vi "Data_filtering_speed_test.vi"() -> ()   [LabVIEW 2018]
uses:
  SubVi's/Controls/CTL_Filter_selector.ctl
  <vilib>/Analysis/NI_AALBase.lvlib
panel:
  out "0th order SG coefficients":dbl[](array[numeric])
  out "subarray":dbl[](array[numeric])
  in  "Filter type 3":u16(ring)=6 items=["None", "Kalman 0.50", "Kalman 0.30", "Kalman 0.12", "Savitzky-Golay 3/5", "Savitzky-Golay 3/11", "Savitzky-Golay 3/31"]
  out "Waveform Chart 3":T1(graph)
  in  "Filter type 2":T2={"Type"=1, "Length"=31, "Order"=3} {"Length" min=5 max=301 step=2; "Order" min=3 max=11 step=2; "Type" items=["None", "Savitzky-Golay"]}
  in  "Filter type":T2={"Type"=1, "Length"=31, "Order"=3} {"Length" min=5 max=301 step=2; "Order" min=3 max=11 step=2; "Type" items=["None", "Savitzky-Golay"]}
  out "standard deviation 2":dbl format="%0.2f"
  out "us per calc 2":dbl format="%0.2f"
  out "Calc time histogram 2":T3(graph)
  out "Waveform Chart 2":cluster{"Filtered sample":dbl, "X1":sgl}(graph)
  out "standard deviation":dbl format="%0.2f"
  out "us per calc":dbl format="%0.2f"
  out "Calc time histogram":T3(graph)
  out "Waveform Chart":cluster{"X1 filtered":dbl, "X1 raw":dbl}(graph)
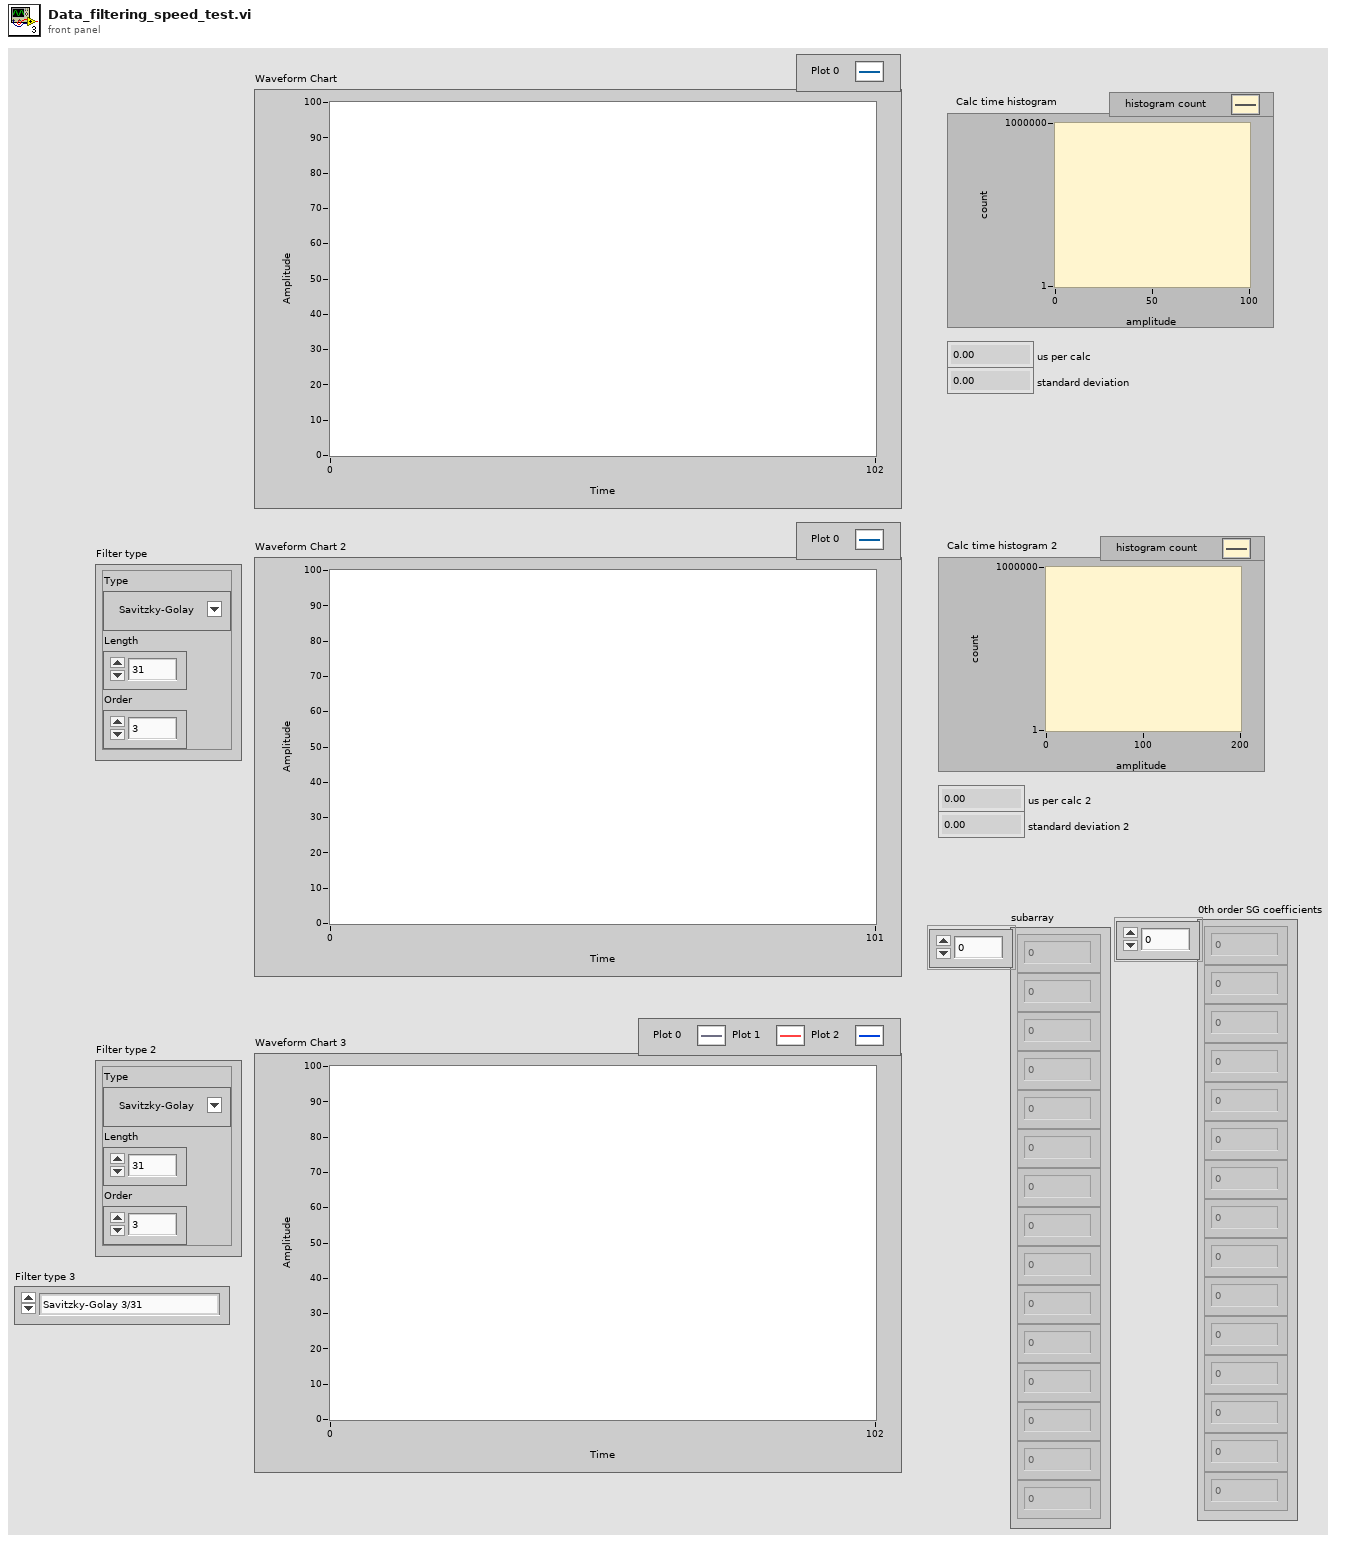
[diagram p1: front panel]
types:
  T1 = cluster{"X1 raw":dbl, "X1 filtered":dbl, "Filtered sample":dbl}
  T2 = typedef "CTL_Filter_selector.ctl" = cluster{"Type":u16, "Length":i32, "Order":i32}
  T3 = cluster{"X Values":dbl[], "Histogram: h(x)":i32[]}
  T4 = cluster{"SG coefficients 3/5":cluster{"0th order SG coefficients":dbl[], "1st order SG coefficients":dbl[]}, "SG coefficients 3/11":cluster{"0th order SG coefficients":dbl[], "1st order SG coefficients":dbl[]}, "SG coefficients 3/31":cluster{"0th order SG coefficients":dbl[], "1st order SG coefficients":dbl[]}, "SG coefficients 3/51":cluster{"0th order SG coefficients":dbl[], "1st order SG coefficients":dbl[]}}
  T5 = cluster{"0th order SG coefficients":dbl[], "1st order SG coefficients":dbl[]}
  T6 = cluster{"ms since ON":u32, "delta time":u32, "X1":sgl, "Y1":sgl, "X2":sgl, "Y2":sgl, "TTL in 1":i16, "TTL in 2":i16, "Frame timestamp":timestamp, "Frame OK":bool}
  T7 = cluster{"Filtered sample":dbl, "Filtered sample":dbl, "Filtered sample":dbl, "Filtered sample":dbl}
  T8 = cluster{"X1 filtered":dbl, "Y1 filtered":dbl, "X2 filtered":dbl, "Y2 filtered":dbl, "X1 raw":dbl, "Y1 raw":dbl, "X2 raw":dbl, "Y2 raw":dbl}
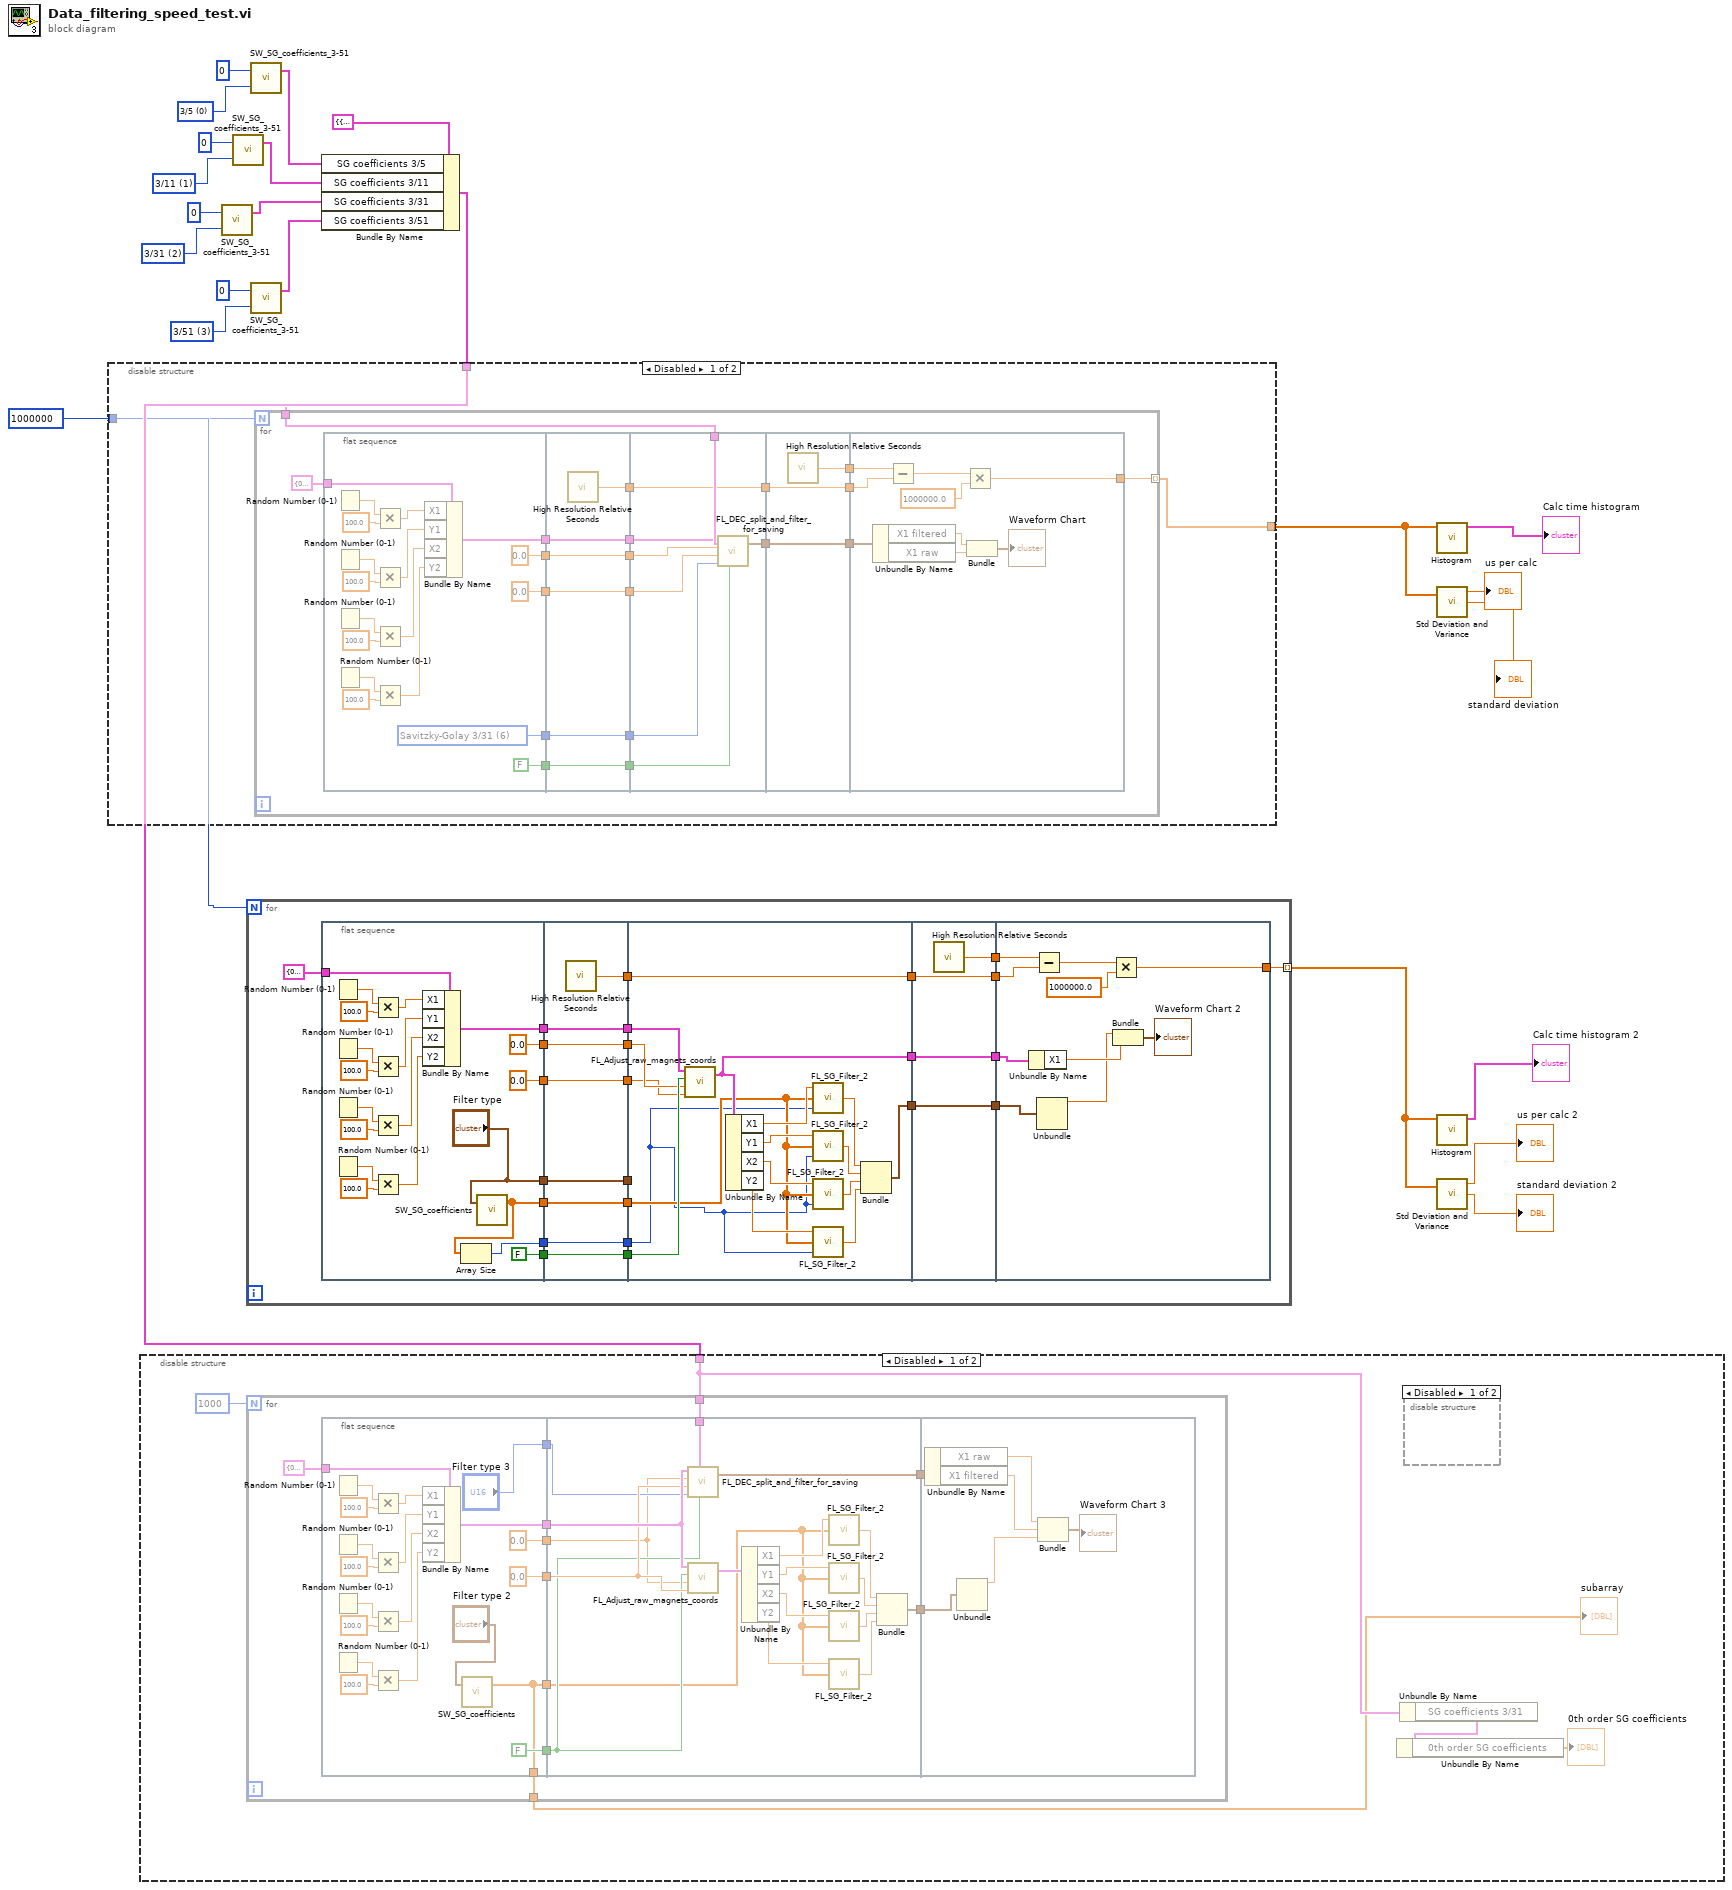
[diagram p0: block diagram]
diagram:
  w9 = 1000000
  w13 = u16 3 items=["3/5", "3/11", "3/31", "3/51"] ("Select filter length")
  w15 = u16 2 items=["3/5", "3/11", "3/31", "3/51"] ("Select filter length")
  w19 = u16 1 items=["3/5", "3/11", "3/31", "3/51"] ("Select filter length")
  w22 = u16 0 items=["3/5", "3/11", "3/31", "3/51"] ("Select filter length")
  n1 = call "SW_SG_coefficients_3-51.vi"("Select filter length"=w15, "Point of interest (can be used for extrapolation)"=0) -> ("SG coefficients"=w14:T5)  [unwired: 1 in]
  n2 = call "SW_SG_coefficients_3-51.vi"("Select filter length"=w19, "Point of interest (can be used for extrapolation)"=0) -> ("SG coefficients"=w17:T5)  [unwired: 1 in]
  n3 = for {
    N: w9 -> [_]
    tunnel: [w34] -> w4 mode=indexing
    n4 = flat-sequence {
      tunnel: T6 {"ms since ON"=0, "delta time"=0, "X1"=0.0, "Y1"=0.0, "X2"=0.0, "Y2"=0.0, "TTL in 1"=0, "TTL in 2"=0, "Frame timestamp"=timestamp(0 s since 1904-01-01), "Frame OK"=FALSE} ("DEC input cluster") -> [w67]
      tunnel: [w54] -> w46
      tunnel: [sgl 0.0 ("Offset V.")] -> w44
      tunnel: [sgl 0.0 ("Offset H.")] -> w42
      tunnel: [FALSE ("Alternative magnets orientation")] -> w40
      tunnel: ["Filter type"] -> w32
      tunnel: [w49] -> w28
      tunnel: [w48] -> w24
      tunnel: w46 -> [w75]
      tunnel: [w75] -> w45
      tunnel: w44 -> [w74]
      tunnel: [w74] -> w43
      tunnel: w42 -> [w73]
      tunnel: [w73] -> w41
      tunnel: w40 -> [w72]
      tunnel: [w72] -> w39
      tunnel: [w71] -> w36
      tunnel: [w70] -> w33
      tunnel: w32 -> [w70]
      tunnel: [w69] -> w29
      tunnel: w28 -> [w69]
      tunnel: [w68] -> w25
      tunnel: w24 -> [w68]
      tunnel: w45 -> [w88]
      tunnel: w43 -> [w90]
      tunnel: w41 -> [w89]
      tunnel: w39 -> [w91]
      tunnel: [w92] -> w37
      tunnel: w36 -> [w92]
      tunnel: w33 -> [_]
      tunnel: [w79] -> w30
      tunnel: w29 -> [w78]
      tunnel: [w77] -> w26
      tunnel: w25 -> [w76]
      tunnel: [w96] -> w38
      tunnel: w37 -> [w96]
      tunnel: [w95] -> w35
      tunnel: [w94] -> w31
      tunnel: w30 -> [w94]
      tunnel: [w93] -> w27
      tunnel: w26 -> [w93]
      tunnel: w38 -> [w104]
      tunnel: w35 -> [w105]
      tunnel: [w102] -> w34
      tunnel: w31 -> [w100]
      tunnel: w27 -> [w99]
      frame #0 {
        n5 = Random Number (0-1)() -> (number: 0 to 1=w66:dbl)
        n6 = Random Number (0-1)() -> (number: 0 to 1=w63:dbl)
        n7 = Random Number (0-1)() -> (number: 0 to 1=w62:dbl)
        n8 = Random Number (0-1)() -> (number: 0 to 1=w59:dbl)
        n9 = Multiply(x=w66, y=100.0) -> (x*y=w58:dbl)
        n10 = Multiply(x=w63, y=100.0) -> (x*y=w57:dbl)
        n11 = Multiply(x=w62, y=100.0) -> (x*y=w56:dbl)
        n12 = Multiply(x=w59, y=100.0) -> (x*y=w55:dbl)
        n13 = Bundle By Name(cluster=w67, "X1"=w58, "Y1"=w57, "X2"=w56, "Y2"=w55) -> (w54:T6)
        n14 = call "SW_SG_coefficients.vi"("Filter parameters"="Filter type") -> ("SG filter coefficients"=w49:dbl[])  [unwired: 2 in]
        n15 = Array Size(array=w49) -> (size(s)=w48:i32)
      }
      frame #1 {
        n16 = call <vilib>:"High Resolution Relative Seconds.vi"() -> ("relative seconds"=w71:dbl)
      }
      frame #2 {
        n17 = call "FL_Adjust_raw_magnets_coords.vi"("Offset H."=w89, "Offset V."=w90, "Alternative magnets orientation"=w91, "DEC cluster in"=w88) -> ("DEC cluster out"=w79:T6)  [unwired: 3 in]
        n18 = Unbundle By Name(w79) -> ("X1"=w87:sgl, "Y1"=w86:sgl, "X2"=w85:sgl, "Y2"=w84:sgl)
        n19 = call "FL_SG_Filter_2.vi"("N samples"=w76, "SG coefficients"=w78, "Input sample"=w87) -> ("Filtered sample"=w83:dbl)
        n20 = call "FL_SG_Filter_2.vi"("N samples"=w76, "SG coefficients"=w78, "Input sample"=w86) -> ("Filtered sample"=w82:dbl)
        n21 = call "FL_SG_Filter_2.vi"("N samples"=w76, "SG coefficients"=w78, "Input sample"=w85) -> ("Filtered sample"=w81:dbl)
        n22 = call "FL_SG_Filter_2.vi"("N samples"=w76, "SG coefficients"=w78, "Input sample"=w84) -> ("Filtered sample"=w80:dbl)
        n23 = Bundle("Filtered sample"=w83, "Filtered sample"=w82, "Filtered sample"=w81, "Filtered sample"=w80) -> (w77:T7)  [unwired: 1 in]
      }
      frame #3 {
        n24 = call <vilib>:"High Resolution Relative Seconds.vi"() -> ("relative seconds"=w95:dbl)
      }
      frame #4 {
        n25 = Unbundle By Name(w100) -> ("X1"=w98:sgl)
        n26 = Subtract(x=w105, y=w104) -> (x-y=w103:dbl)
        n27 = Unbundle(w99) -> ("Filtered sample"=w97:dbl)  [unwired: 3 out]
        n28 = Multiply(x=w103, y=1000000.0) -> (x*y=w102:dbl)
        n29 = Bundle("Filtered sample"=w97, "X1"=w98) -> (→"Waveform Chart 2":cluster{"Filtered sample":dbl, "X1":sgl})  [unwired: 1 in]
      }
    }
  }
  n30 = call "SW_SG_coefficients_3-51.vi"("Select filter length"=w22, "Point of interest (can be used for extrapolation)"=0) -> ("SG coefficients"=w20:T5)  [unwired: 1 in]
  n31 = call "SW_SG_coefficients_3-51.vi"("Select filter length"=w13, "Point of interest (can be used for extrapolation)"=0) -> ("SG coefficients"=w11:T5)  [unwired: 1 in]
  n32 = Bundle By Name(cluster=T4 {"SG coefficients 3/5"={"0th order SG coefficients"=[], "1st order SG coefficients"=[]}, "SG coefficients 3/11"={"0th order SG coefficients"=[], "1st order SG coefficients"=[]}, "SG coefficients 3/31"={"0th order SG coefficients"=[], "1st order SG coefficients"=[]}, "SG coefficients 3/51"={"0th order SG coefficients"=[], "1st order SG coefficients"=[]}} ("Input cluster of SG coefficients"), "SG coefficients 3/5"=w20, "SG coefficients 3/11"=w17, "SG coefficients 3/31"=w14, "SG coefficients 3/51"=w11) -> (w10:T4)
  n33 = disable-structure shown="Disabled" {
    disable-tunnel: w10 -> [w109 _]
    disable-tunnel: w9 -> [w108 _]
    disable-tunnel: [w107 _] -> w5
    frame Disabled {
      n34 = for {
        N: w108 -> [_]
        tunnel: w109 -> [w127]
        tunnel: [w110] -> w107 mode=indexing
        n35 = flat-sequence {
          tunnel: T6 {"ms since ON"=0, "delta time"=0, "X1"=0.0, "Y1"=0.0, "X2"=0.0, "Y2"=0.0, "TTL in 1"=0, "TTL in 2"=0, "Frame timestamp"=timestamp(0 s since 1904-01-01), "Frame OK"=FALSE} ("DEC input cluster") -> [w146]
          tunnel: [w133] -> w126
          tunnel: [sgl 0.0 ("Offset V.")] -> w124
          tunnel: [sgl 0.0 ("Offset H.")] -> w122
          tunnel: [w130] -> w120
          tunnel: [FALSE ("Alternative magnets orientation")] -> w118
          tunnel: w126 -> [w152]
          tunnel: [w152] -> w125
          tunnel: w124 -> [w151]
          tunnel: [w151] -> w123
          tunnel: w122 -> [w150]
          tunnel: [w150] -> w121
          tunnel: w120 -> [w149]
          tunnel: [w149] -> w119
          tunnel: w118 -> [w148]
          tunnel: [w148] -> w117
          tunnel: [w147] -> w112
          tunnel: w127 -> [w160]
          tunnel: w125 -> [w159]
          tunnel: w123 -> [w158]
          tunnel: w121 -> [w157]
          tunnel: w119 -> [w156]
          tunnel: w117 -> [w155]
          tunnel: [w154] -> w116
          tunnel: [w153] -> w113
          tunnel: w112 -> [w153]
          tunnel: w116 -> [w163]
          tunnel: [w163] -> w115
          tunnel: [w162] -> w114
          tunnel: w113 -> [w162]
          tunnel: [w161] -> w111
          tunnel: w115 -> [w172]
          tunnel: w114 -> [w167]
          tunnel: w111 -> [w168]
          tunnel: [w165] -> w110
          frame #0 {
            w130 = u16 6 items=["None", "Kalman 0.50", "Kalman 0.30", "Kalman 0.12", "Savitzky-Golay 3/5", "Savitzky-Golay 3/11", "Savitzky-Golay 3/31"] ("Filter type")
            n36 = Random Number (0-1)() -> (number: 0 to 1=w145:dbl)
            n37 = Random Number (0-1)() -> (number: 0 to 1=w142:dbl)
            n38 = Random Number (0-1)() -> (number: 0 to 1=w141:dbl)
            n39 = Random Number (0-1)() -> (number: 0 to 1=w138:dbl)
            n40 = Multiply(x=w145, y=100.0) -> (x*y=w137:dbl)
            n41 = Multiply(x=w142, y=100.0) -> (x*y=w136:dbl)
            n42 = Multiply(x=w141, y=100.0) -> (x*y=w135:dbl)
            n43 = Multiply(x=w138, y=100.0) -> (x*y=w134:dbl)
            n44 = Bundle By Name(cluster=w146, "X1"=w137, "Y1"=w136, "X2"=w135, "Y2"=w134) -> (w133:T6)
          }
          frame #1 {
            n45 = call <vilib>:"High Resolution Relative Seconds.vi"() -> ("relative seconds"=w147:dbl)
          }
          frame #2 {
            n46 = call "FL_DEC_split_and_filter_for_saving.vi"("Alternative magnets orientation"=w155, "Input cluster of SG coefficients"=w160, "Filter type"=w156, "Offset H."=w157, "Offset V."=w158, "DEC input cluster"=w159) -> ("Magnets coords"=w154:T8)  [unwired: 1 in]
          }
          frame #3 {
            n47 = call <vilib>:"High Resolution Relative Seconds.vi"() -> ("relative seconds"=w161:dbl)
          }
          frame #4 {
            n48 = Unbundle By Name(w172) -> ("X1 filtered"=w171:dbl, "X1 raw"=w170:dbl)
            n49 = Subtract(x=w168, y=w167) -> (x-y=w166:dbl)
            n50 = Multiply(x=w166, y=1000000.0) -> (x*y=w165:dbl)
            n51 = Bundle("X1 filtered"=w171, "X1 raw"=w170) -> (→"Waveform Chart":cluster{"X1 filtered":dbl, "X1 raw":dbl})  [unwired: 1 in]
          }
        }
      }
    }
    frame Enabled {
    }
  }
  n52 = disable-structure shown="Disabled" {
    disable-tunnel: w10 -> [w176 _]
    frame Disabled {
      n53 = for {
        N: 1000 -> [_]
        tunnel: w176 -> [w182]
        tunnel: [w180] -> w173
        n54 = flat-sequence {
          tunnel: T6 {"ms since ON"=0, "delta time"=0, "X1"=0.0, "Y1"=0.0, "X2"=0.0, "Y2"=0.0, "TTL in 1"=0, "TTL in 2"=0, "Frame timestamp"=timestamp(0 s since 1904-01-01), "Frame OK"=FALSE} ("DEC input cluster") -> [w208]
          tunnel: [w195] -> w187
          tunnel: [sgl 0.0 ("Offset V.")] -> w186
          tunnel: [sgl 0.0 ("Offset H.")] -> w185
          tunnel: [FALSE ("Alternative magnets orientation")] -> w184
          tunnel: ["Filter type 3"] -> w183
          tunnel: [w189] -> w180
          tunnel: [w189] -> w179
          tunnel: w187 -> [w226]
          tunnel: w186 -> [w218]
          tunnel: w185 -> [w225]
          tunnel: w184 -> [w222]
          tunnel: w183 -> [w224]
          tunnel: w182 -> [w223]
          tunnel: [w221] -> w181
          tunnel: w179 -> [w214]
          tunnel: [w209] -> w178
          tunnel: w181 -> [w231]
          tunnel: w178 -> [w228]
          frame #0 {
            n55 = Random Number (0-1)() -> (number: 0 to 1=w207:dbl)
            n56 = Random Number (0-1)() -> (number: 0 to 1=w204:dbl)
            n57 = Random Number (0-1)() -> (number: 0 to 1=w203:dbl)
            n58 = Random Number (0-1)() -> (number: 0 to 1=w200:dbl)
            n59 = Multiply(x=w207, y=100.0) -> (x*y=w199:dbl)
            n60 = Multiply(x=w204, y=100.0) -> (x*y=w198:dbl)
            n61 = Multiply(x=w203, y=100.0) -> (x*y=w197:dbl)
            n62 = Multiply(x=w200, y=100.0) -> (x*y=w196:dbl)
            n63 = Bundle By Name(cluster=w208, "X1"=w199, "Y1"=w198, "X2"=w197, "Y2"=w196) -> (w195:T6)
            n64 = call "SW_SG_coefficients.vi"("Filter parameters"="Filter type 2") -> ("SG filter coefficients"=w189:dbl[])  [unwired: 2 in]
          }
          frame #1 {
            n65 = call "FL_DEC_split_and_filter_for_saving.vi"("Alternative magnets orientation"=w222, "Input cluster of SG coefficients"=w223, "Filter type"=w224, "Offset H."=w225, "Offset V."=w218, "DEC input cluster"=w226) -> ("Magnets coords"=w221:T8)  [unwired: 1 in]
            n66 = call "FL_Adjust_raw_magnets_coords.vi"("Offset H."=w225, "Offset V."=w218, "Alternative magnets orientation"=w222, "DEC cluster in"=w226) -> ("DEC cluster out"=w220:T6)  [unwired: 3 in]
            n67 = Unbundle By Name(w220) -> ("X1"=w219:sgl, "Y1"=w217:sgl, "X2"=w216:sgl, "Y2"=w215:sgl)
            n68 = call "FL_SG_Filter_2.vi"("SG coefficients"=w214, "Input sample"=w219) -> ("Filtered sample"=w213:dbl)  [unwired: 1 in]
            n69 = call "FL_SG_Filter_2.vi"("SG coefficients"=w214, "Input sample"=w217) -> ("Filtered sample"=w212:dbl)  [unwired: 1 in]
            n70 = call "FL_SG_Filter_2.vi"("SG coefficients"=w214, "Input sample"=w216) -> ("Filtered sample"=w211:dbl)  [unwired: 1 in]
            n71 = call "FL_SG_Filter_2.vi"("SG coefficients"=w214, "Input sample"=w215) -> ("Filtered sample"=w210:dbl)  [unwired: 1 in]
            n72 = Bundle("Filtered sample"=w213, "Filtered sample"=w212, "Filtered sample"=w211, "Filtered sample"=w210) -> (w209:T7)  [unwired: 1 in]
          }
          frame #2 {
            n73 = Unbundle By Name(w231) -> ("X1 raw"=w230:dbl, "X1 filtered"=w229:dbl)
            n74 = Unbundle(w228) -> ("Filtered sample"=w227:dbl)  [unwired: 3 out]
            n75 = Bundle("X1 raw"=w230, "X1 filtered"=w229, "Filtered sample"=w227) -> (→"Waveform Chart 3":T1)  [unwired: 1 in]
          }
        }
      }
      "subarray" <- w173
      n76 = Unbundle By Name(w176) -> ("SG coefficients 3/31"=w175:T5)
      n77 = Unbundle By Name(w175) -> ("0th order SG coefficients"=→"0th order SG coefficients":dbl[])
      n78 = disable-structure shown="Disabled" {
        frame Disabled {
        }
        frame Enabled {
        }
      }
    }
    frame Enabled {
    }
  }
  n79 = call <vilib>:"Histogram.vi"("X"=w5) -> ("Histogram Graph"=→"Calc time histogram":T3)  [unwired: 7 in, 3 out]
  n80 = call <vilib>:"Std Deviation and Variance.vi"("X"=w5) -> ("mean"=→"us per calc":dbl, "standard deviation"=→"standard deviation":dbl)  [unwired: 1 in, 1 out]
  n81 = call <vilib>:"Histogram.vi"("X"=w4) -> ("Histogram Graph"=→"Calc time histogram 2":T3)  [unwired: 7 in, 3 out]
  n82 = call <vilib>:"Std Deviation and Variance.vi"("X"=w4) -> ("mean"=→"us per calc 2":dbl, "standard deviation"=→"standard deviation 2":dbl)  [unwired: 1 in, 1 out]
